vi "Serial_Write_Read_Event_xbox_Polling.vi"() -> ()   [LabVIEW 2023]
uses:
  <vilib>/MakerHub/Xbox-One-Controller/Private/Type Defs/Indicators/Controller.ctl
  <vilib>/MakerHub/Xbox-One-Controller/Private/Type Defs/Indicators/A.ctl
  <vilib>/MakerHub/Xbox-One-Controller/Private/Type Defs/Indicators/B.ctl
  <vilib>/MakerHub/Xbox-One-Controller/Private/Type Defs/Indicators/X.ctl
  <vilib>/MakerHub/Xbox-One-Controller/Private/Type Defs/Indicators/Y.ctl
  <vilib>/MakerHub/Xbox-One-Controller/Private/Type Defs/Indicators/Left Bumper.ctl
  <vilib>/MakerHub/Xbox-One-Controller/Private/Type Defs/Indicators/Right Bumper.ctl
  <vilib>/MakerHub/Xbox-One-Controller/Private/Type Defs/Indicators/View.ctl
  <vilib>/MakerHub/Xbox-One-Controller/Private/Type Defs/Indicators/Menu.ctl
  <vilib>/MakerHub/Xbox-One-Controller/Private/Type Defs/Indicators/Thumbstick_Analog.ctl
  <vilib>/MakerHub/Xbox-One-Controller/Private/Type Defs/Indicators/Slider.ctl
  <vilib>/MakerHub/Xbox-One-Controller/Private/Type Defs/Indicators/DPad.ctl
  <vilib>/MakerHub/Xbox-One-Controller/Public/Open First Controller.vi
  <vilib>/Instr/_visa.llb/VISA Configure Serial Port (Instr).vi
  <vilib>/MakerHub/Xbox-One-Controller/LMH-Xbox-One-Controller.lvlib
panel:
  out "X Axis Right":i32 format="%#.0f"
  out "Y Axis Left":i32
  out "Error Out":errorcluster
  in  "byte count\nRead":u32=80
  out "Serial Buffer (Read)":string
  in  "Left Stick":u32(slide)=50 scale=0.0..100.0
  out "Loop Count":i32
  out "Panel Outputs\nActive":bool
  in  "Right Bumper":T1 caption="Blank Button"
  in  "Left Bumper":T2 caption="Blank Button"
  in  "Menu Button":T3 caption="Blank Button"
  in  "View Button":T4 caption="Blank Button"
  in  "Y":T5 caption="Blank Button"
  in  "X":T6 caption="Blank Button"
  in  "B":T7 caption="Blank Button"
  in  "A":T8 caption="Blank Button"
  in  "Right Stick":u32(slide)=50 scale=0.1..100.0
  in  "Panel Buttons / Xbox Buttons":bool
  out "Controller":T9={"A Button"=FALSE, "B Button"=FALSE, "X Button"=FALSE, "Y Button"=FALSE, "Left Bumper"=FALSE, "Right Bumper"=FALSE, "View Button"=FALSE, "Menu Button"=FALSE, "Left Stick"={[], []}, "Right Stick"={[], []}, "Trigger"=0, "D-Pad"=5} {"Trigger" scale=32767.0..-32768.0}
  out "error out":errorcluster
  in  "error in (no error)":errorcluster
  in  "Loop Timer ms":u32=100 min=10
  out "Concatenated \nString For Transmission":string
  in  "VISA resource name":refnum<visa-resource-name>="COM8"
  out "byte count Sent":u32
  out "Controller Outputs\nActive":bool
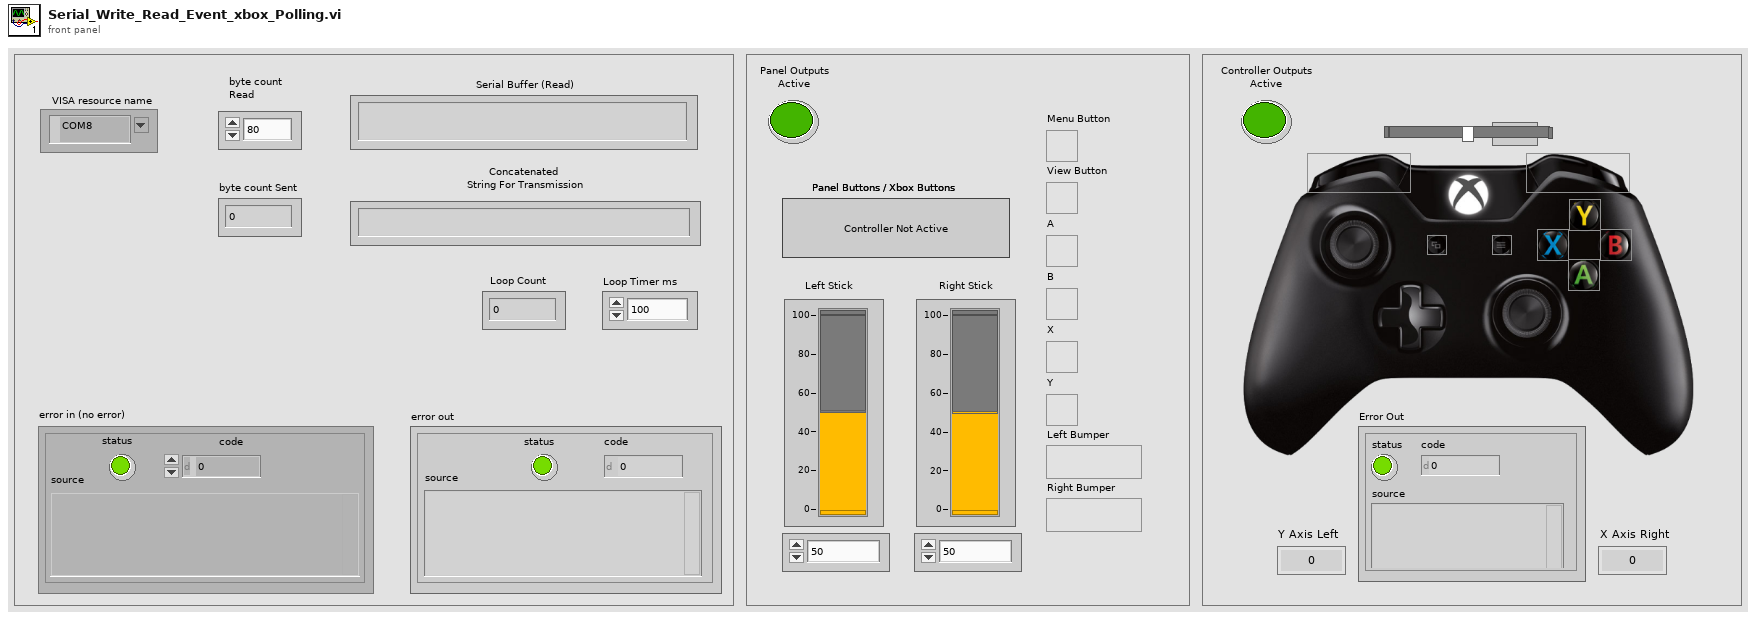
[diagram p1: front panel]
types:
  T1 = typedef "LMH-Xbox-One-Controller.lvlib/Right Bumper.ctl" = bool
  T2 = typedef "LMH-Xbox-One-Controller.lvlib/Left Bumper.ctl" = bool
  T3 = typedef "LMH-Xbox-One-Controller.lvlib/Menu.ctl" = bool
  T4 = typedef "LMH-Xbox-One-Controller.lvlib/View.ctl" = bool
  T5 = typedef "LMH-Xbox-One-Controller.lvlib/Y.ctl" = bool
  T6 = typedef "LMH-Xbox-One-Controller.lvlib/X.ctl" = bool
  T7 = typedef "LMH-Xbox-One-Controller.lvlib/B.ctl" = bool
  T8 = typedef "LMH-Xbox-One-Controller.lvlib/A.ctl" = bool
  T9 = typedef "LMH-Xbox-One-Controller.lvlib/Controller.ctl" = cluster{"A Button":T8, "B Button":T7, "X Button":T6, "Y Button":T5, "Left Bumper":T2, "Right Bumper":T1, "View Button":T4, "Menu Button":T3, "Left Stick":T10, "Right Stick":T10, "Trigger":T11, "D-Pad":T12}
  T10 = typedef "LMH-Xbox-One-Controller.lvlib/Thumbstick_Analog.ctl" = cluster{i32[], i32[]}
  T11 = typedef "LMH-Xbox-One-Controller.lvlib/Slider.ctl" = i32
  T12 = typedef "LMH-Xbox-One-Controller.lvlib/DPad.ctl" = u16
  T13 = typedef "LMH-Xbox-One-Controller.lvlib/Xbox One Controller Ref.ctl" = cluster{"Controller Ref":refnum<k1>, "Event Refnum":refnum<event-registration>, "Worker Ref":refnum<vi>}
  T14 = typedef "LMH-Xbox-One-Controller.lvlib/All Axis Data.ctl" = cluster{"Left Stick":cluster{"X Axis":i32, "Y Axis":i32}, "Right Stick":cluster{"X Axis":i32, "Y Axis":i32}, "Triggers":i32, "D-Pad":T15}
  T15 = typedef "LMH-Xbox-One-Controller.lvlib/DPad Enum.ctl" = enum16{"Idle", "Up", "Up / Right", "Right", "Down / Right", "Down", "Down / Left", "Left", "Up / Left"}
  T16 = typedef "LMH-Xbox-One-Controller.lvlib/All Buttons Visual.ctl" = cluster{"A":T8, "B":T7, "X":T6, "Y":T5, "Left Bumper":T2, "Right Bumper":T1, "View Button":T4, "Menu Button":T3, "Left Stick":T17, "Right Stick":T17}
  T17 = typedef "LMH-Xbox-One-Controller.lvlib/Thumbstick.ctl" = bool
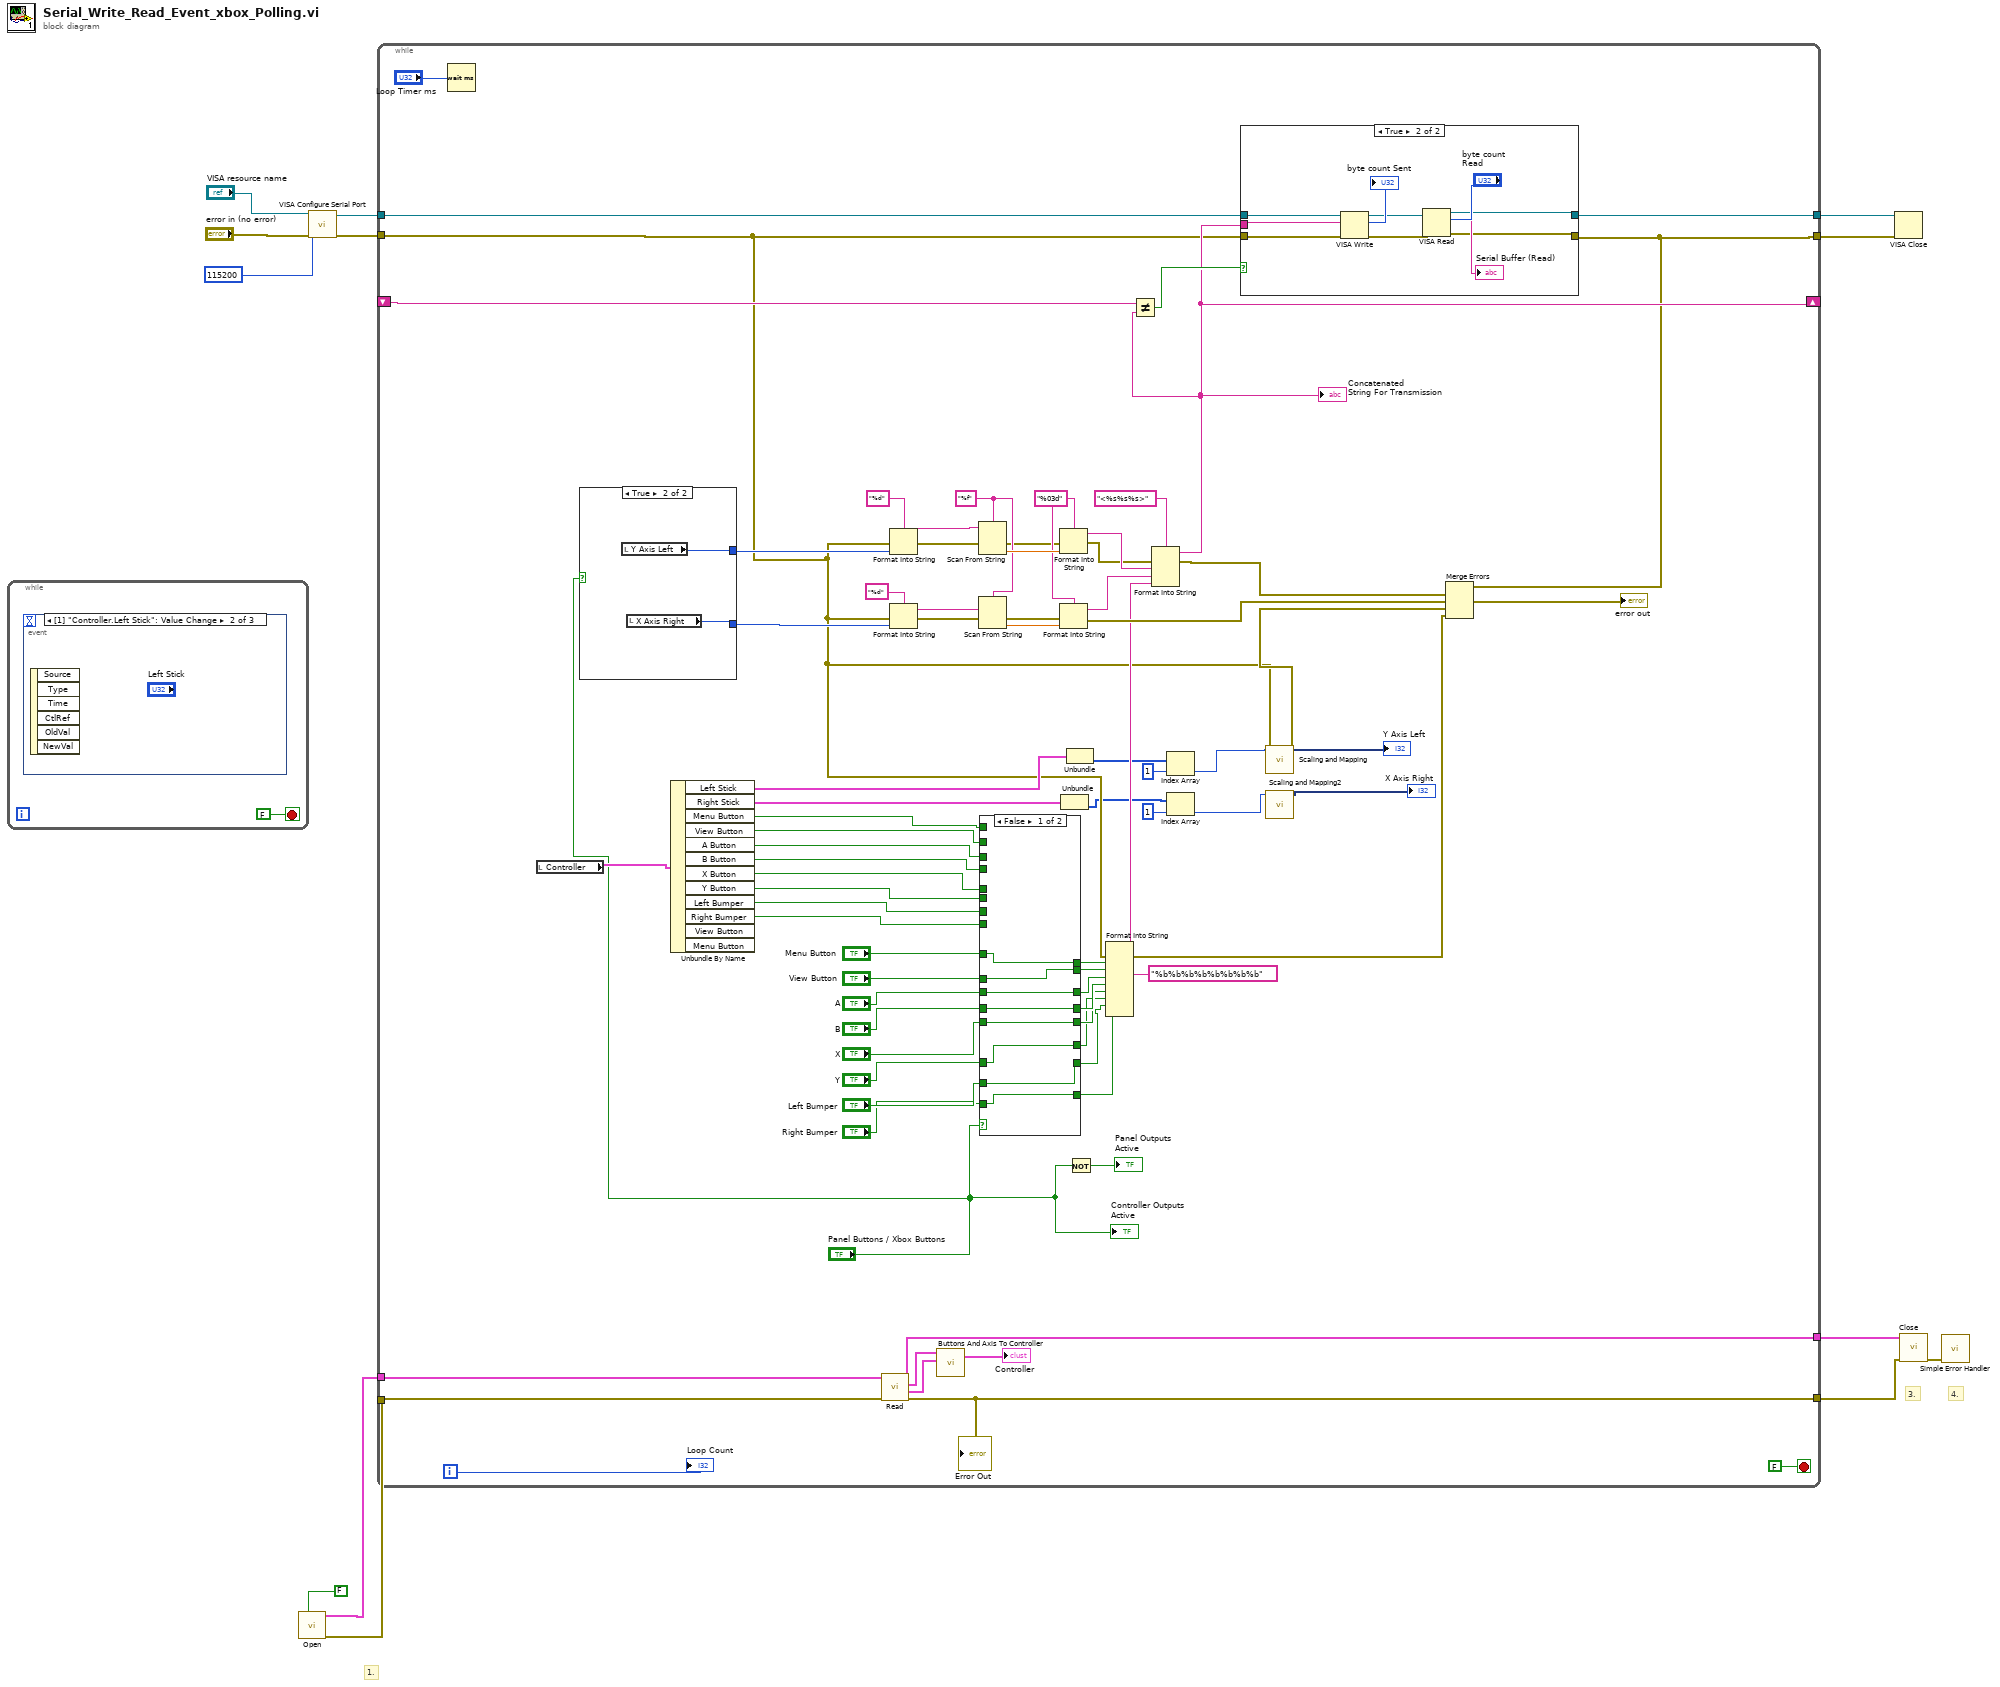
[diagram p0: block diagram]
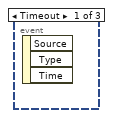
[diagram p2: hidden frame]
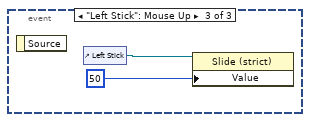
[diagram p3: hidden frame]
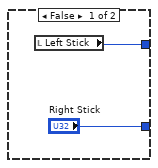
[diagram p4: hidden frame]
diagram:
  # "4."
  # "3."
  # "1."
  n1 = while {
    stop <- FALSE stop-if-true
    n2 = event shown="[1] \"Controller.Left Stick\": Value Change" {
      selector: _ -> [_ _ _]
      dyn-events: _ -> [_ _ _]
      timeout: _ -> [_ _ _]
      event Timeout {
        n3 = event-data() -> ()  [unwired: 1 in, 3 out]
      }
      event Value Change {
        n4 = event-data() -> ()  [unwired: 1 in, 6 out]
      }
      event "Left Stick": Mouse Up {
        n5 = event-data() -> ()  [unwired: 1 in, 1 out]
        n6 = control-ref of="Left Stick"() -> (w16:refnum<vi>)
        n7 = property class="Slide (strict)"(reference=w16, "Value"=u32 50) -> ()  [unwired: 1 in, 2 out]
      }
    }
  }
  n8 = call-poly <vilib>:"Open.vi"("Enable Events (T)"=FALSE) -> ("Error Out"=w3:errorcluster, "Xbox One Controller"=w4:T13)  [unwired: 8 in, 1 out]
  n9 = call-poly "VISA Configure Serial Port"("VISA resource name"="VISA resource name", "baud rate (9600)"=u32 115200, "error in (no error)"="error in (no error)") -> ("VISA resource name out"=w5:refnum<visa-resource-name>, "error out"=w8:errorcluster)  [unwired: 11 in]
  n10 = while {
    tunnel: w8 -> [w33]
    tunnel: [w34] -> w7
    tunnel: [w35] -> w6
    tunnel: w5 -> [w32]
    shift-right: [w36] -> _
    shift-left: _ -> [w38]
    tunnel: w4 -> [w28]
    tunnel: w3 -> [w27]
    tunnel: [w26] -> w2
    tunnel: [w25] -> w1
    i -> [w44]
    stop <- FALSE stop-if-true
    w88 = "%f" ("format string")
    w90 = "%03d" ("format string")
    n11 = Wait (ms)(milliseconds to wait="Loop Timer ms") -> ()  [unwired: 1 out]
    n12 = local read "Controller"() -> (w43:T9)
    n13 = case shown="True" "Panel Buttons / Xbox Buttons" {
      tunnel: ["Right Stick" w98] -> w46
      tunnel: [w96 w99] -> w40
      frame False {
        n14 = local read "Left Stick"() -> (w96:u32)
      }
      frame True {
        n15 = local read "Y Axis Left"() -> (w99:i32)
        n16 = local read "X Axis Right"() -> (w98:i32)
      }
    }
    n17 = Unbundle By Name(w43) -> ("Left Stick"=w76:T10, "Right Stick"=w75:T10, "Menu Button"=w54:T3, "View Button"=w53:T4, "A Button"=w52:T8, "B Button"=w51:T7, "X Button"=w50:T6, "Y Button"=w49:T5, "Left Bumper"=w48:T2, "Right Bumper"=w47:T1)  [unwired: 2 out]
    n18 = call <vilib>:"Read.vi"("Error In"=w27, "Xbox One Controller Ref"=w28) -> ("Error Out"=w26:errorcluster, "All Axis"=w30:T14, "Buttons"=w29:T16, "Xbox One Controller Ref"=w25:T13)  [unwired: 6 in]
    "Error Out" <- w26
    n19 = Format Into String(format string="%d", error in=w33, w40) -> (resulting string=w94:string, error out=w84:errorcluster)  [unwired: 1 in]
    n20 = Format Into String(format string="%d", error in=w33, w46) -> (resulting string=w89:string, error out=w81:errorcluster)  [unwired: 1 in]
    n21 = call <vilib>:"Buttons And Axis To Controller.vi"("All Axis"=w30, "Buttons"=w29) -> ("Controller"=→"Controller":T9)  [unwired: 5 in]
    n22 = Scan From String(format string=w88, input string=w94, error in=w84) -> (error out=w83:errorcluster, output 1=w95:dbl)  [unwired: 2 in, 2 out]
    n23 = Scan From String(format string=w88, input string=w89, error in=w81) -> (error out=w80:errorcluster, output 1=w85:dbl)  [unwired: 2 in, 2 out]
    n24 = case shown="False" "Panel Buttons / Xbox Buttons" {
      tunnel: "Menu Button" -> [w119 _]
      tunnel: [w119 w127] -> w69
      tunnel: "View Button" -> [w118 _]
      tunnel: [w118 w126] -> w67
      tunnel: "A" -> [w117 _]
      tunnel: [w117 w125] -> w65
      tunnel: "B" -> [w116 _]
      tunnel: "X" -> [w115 _]
      tunnel: "Y" -> [w114 _]
      tunnel: "Left Bumper" -> [w113 _]
      tunnel: "Right Bumper" -> [w112 _]
      tunnel: [w116 w124] -> w59
      tunnel: [w115 w123] -> w58
      tunnel: [w114 w122] -> w57
      tunnel: [w113 w121] -> w56
      tunnel: [w112 w120] -> w55
      tunnel: w54 -> [_ w127]
      tunnel: w53 -> [_ w126]
      tunnel: w52 -> [_ w125]
      tunnel: w51 -> [_ w124]
      tunnel: w50 -> [_ w123]
      tunnel: w49 -> [_ w122]
      tunnel: w48 -> [_ w121]
      tunnel: w47 -> [_ w120]
      frame False {
      }
      frame True {
      }
    }
    n25 = Format Into String(format string=w90, error in=w83, w95) -> (resulting string=w93:string, error out=w82:errorcluster)  [unwired: 1 in]
    n26 = Format Into String(format string=w90, error in=w80, w85) -> (resulting string=w91:string, error out=w78:errorcluster)  [unwired: 1 in]
    n27 = Unbundle(w75) -> (w21:i32[])  [unwired: 1 out]
    n28 = Unbundle(w76) -> (w24:i32[])  [unwired: 1 out]
    n29 = Not(x="Panel Buttons / Xbox Buttons") -> (.not. x?=→"Panel Outputs\nActive":bool)
    n30 = Format Into String(format string="%b%b%b%b%b%b%b%b", error in=w33, w69, w67, w65, w59, w58, w57, w56, w55) -> (resulting string=w72:string, error out=w45:errorcluster)  [unwired: 1 in]
    n31 = Format Into String(format string="<%s%s%s>", error in=w82, w93, w91, w72) -> (resulting string=w36:string, error out=w79:errorcluster)  [unwired: 1 in]
    "Concatenated \nString For Transmission" <- w36
    n32 = Not Equal?(x=w38, y=w36) -> (x != y?=w37:bool)
    n33 = Index Array(array=w24, index=1) -> (element=w22:i32)
    n34 = Index Array(array=w21, index=1) -> (element=w19:i32)
    n35 = case shown="True" w37 {
      tunnel: w33 -> [w100 w110]
      tunnel: w32 -> [w101 w109]
      tunnel: w36 -> [_ w108]
      tunnel: [w100 w102] -> w34
      tunnel: [w101 w103] -> w35
      frame False {
      }
      frame True {
        n36 = VISA Write(VISA resource name=w109, write buffer=w108, error in (no error)=w110) -> (VISA resource name out=w105:refnum<visa-resource-name>, return count=→"byte count Sent":u32, error out=w104:errorcluster)
        n37 = VISA Read(VISA resource name=w105, byte count="byte count\nRead", error in (no error)=w104) -> (VISA resource name out=w103:refnum<visa-resource-name>, read buffer=→"Serial Buffer (Read)":string, error out=w102:errorcluster)  [unwired: 1 out]
      }
    }
    n38 = call "Scaling and Mapping"("error in (no error)"=w33, "Signals"=w22) -> ("error out"=w73:errorcluster, "Scaled Signals"=→"Y Axis Left":dynamicdata)  [unwired: 8 in]
    n39 = call "Scaling and Mapping2"("Signals"=w19) -> ("Scaled Signals"=→"X Axis Right":dynamicdata)  [unwired: 9 in, 1 out]
    n40 = Merge Errors(w34, w79, w78, w73, w45) -> (→"error out":errorcluster)
    "Controller Outputs\nActive" <- "Panel Buttons / Xbox Buttons"
    "Loop Count" <- w44
  }
  n41 = VISA Close(VISA resource name=w6, error in (no error)=w7) -> ()  [unwired: 1 out]
  n42 = call <vilib>:"Close.vi"("Error In"=w2, "Xbox One Controller Ref"=w1) -> ("Error Out"=w11:errorcluster)  [unwired: 9 in]
  n43 = call <vilib>:"Simple Error Handler.vi"("error in (no error)"=w11) -> ()  [unwired: 4 in, 5 out]
